vi "Test_PublishI32_SubBeforePub_OK.vi"(8 "error in (no error)":errorcluster, 11 "TestMediator In":refnum<class "TestMediationSemantics.lvclass">) -> (0 "error out":errorcluster, 3 "TestMediator Out":refnum<class "TestMediationSemantics.lvclass">)   [LabVIEW 2017, in "TestMediationSemantics.lvclass"]
uses:
  TestMediationSemantics.lvclass
  Source/Framework/Mediator/Mediator/Mediator.lvclass
  C:/Program Files (x86)/National Instruments/LabVIEW 2017/vi.lib/ActorFramework/Actor/Actor.lvclass
  Source/Framework/IMediator/PublishRequest/PublishRequest.lvclass/PublishRequest.ctl
  Source/Framework/SubscriptionPolicy/BasicSubscription/BasicSubscription.lvclass/BasicSubscription.ctl
  Source/Framework/IMediator/SubscriptionRequest/SubscriptionRequest.lvclass/SubscriptionRequest.ctl
  Source/Framework/IMediator/IMediator Messages/Subscribe Msg/Subscribe Msg.lvclass/Subscribe Msg.ctl
  <vilib>/ActorFramework/Message Enqueuer/Message Enqueuer.lvclass/Message Enqueuer.ctl
  Source/Framework/IMediator/IMediator Messages/Publish Msg/Publish Msg.lvclass/Publish Msg.ctl
  gpm_packages/@cs/transport/Source/Concrete/QueueTransport/QueueTransport.lvclass/QueueTransport.ctl
  <vilib>/ActorFramework/Message Enqueuer/Enqueue.vi
  Source/Framework/SubscriptionPolicy/BasicSubscription/BasicSubscription.lvclass
  C:/Git/mva-framework/Source/Framework/IMediator/ISubscriptionPolicy/ISubscriptionPolicy.lvclass
  gpm_packages/@cs/transport/Source/Concrete/QueueTransport/QueueTransport.lvclass
  C:/Git/mva-framework/gpm_packages/@cs/transport/Source/ITransport/ITransport.lvclass
  Source/Framework/IMediator/IMediator Messages/Subscribe Msg/Subscribe Msg.lvclass
  C:/Program Files (x86)/National Instruments/LabVIEW 2017/vi.lib/ActorFramework/Message/Message.lvclass
  Source/Framework/IMediator/IMediator Messages/Publish Msg/Publish Msg.lvclass
  <vilib>/ActorFramework/Stop Msg/Stop Msg.lvclass
  <vilib>/ActorFramework/Message Priority Queue/Priority Enqueue.vi
  <vilib>/Utility/error.llb/Error Cluster From Error Code.vi
  Source/Framework/IMediator/SubscriptionRequest/SubscriptionRequest.lvclass
  Source/Framework/IMediator/PublishRequest/PublishRequest.lvclass
  <vilib>/ActorFramework/Actor/Actor.lvclass
  Source/Framework/IMediator/ISubscriptionPolicy/ISubscriptionPolicy.lvclass
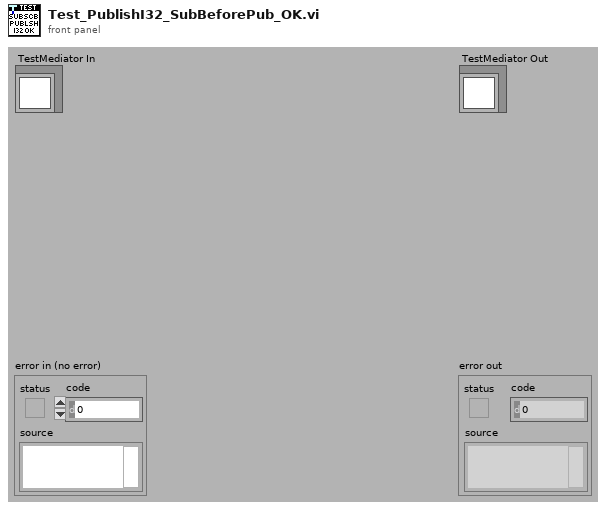
[diagram p1: front panel]
types:
  T1 = typedef "IMediator.lvlib/ISubscriptionPolicy.lvclass/ISubscriptionPolicy Reference.ctl" = refnum<data-value>
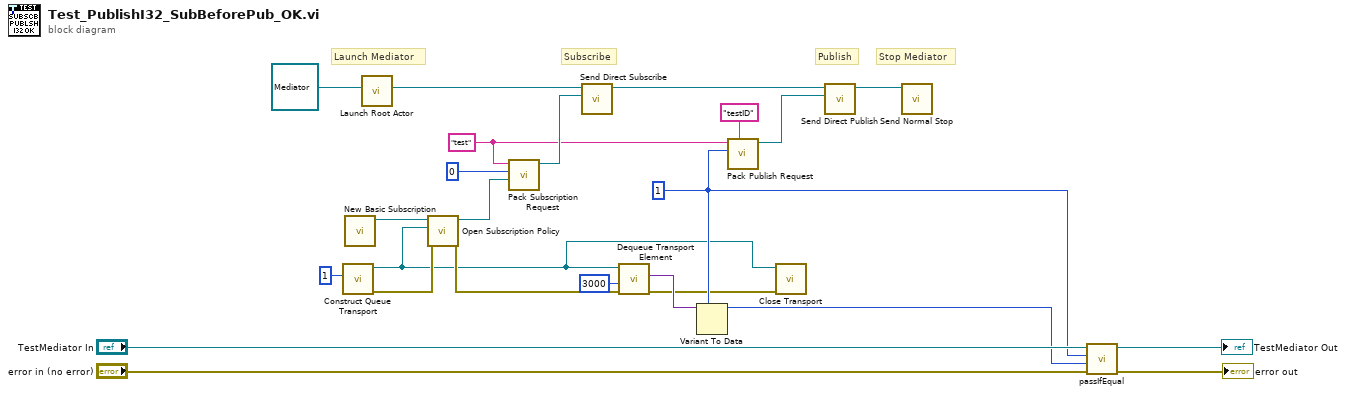
[diagram p0: block diagram]
diagram:
  w5 = "test" ("Datum Name")
  w4 = 1
  # "Launch Mediator"
  # "Stop Mediator"
  # "Subscribe"
  # "Publish"
  n1 = call "Construct Queue Transport.vi"("Max Queue Size (-1)"=1) -> ("error out"=w15:errorcluster, "QueueTransport"=w2:refnum<class "QueueTransport.lvclass">)  [unwired: 9 in]
  n2 = call "New Basic Subscription.vi"() -> ("BasicSubscription Out"=w11:refnum<class "BasicSubscription.lvclass">)  [unwired: 11 in]
  n3 = call <vilib>:"Launch Root Actor.vi"("Actor"=refnum<class "Mediator.lvclass"> refnum ("Mediator.lvlib:Mediator.lvclass")) -> ("Actor's Enqueuer"=w8:refnum<class "Message Enqueuer.lvclass">)  [unwired: 9 in, 1 out]
  n4 = call "Open Subscription Policy.vi"("error in (no error)"=w15, "Transport"=w2, "SubscriptionPolicy"=w11) -> ("error out"=w14:errorcluster, "Subscription Policy"=w7:T1)  [unwired: 7 in]
  n5 = call "Pack Subscription Request.vi"("Subscription Policy"=w7, "Type"=0, "Datum Name"=w5) -> ("SubscriptionRequest"=w19:refnum<class "SubscriptionRequest.lvclass">)  [unwired: 8 in]
  n6 = call "Send Direct Subscribe.vi"("Subscription Request"=w19, "Message Enqueuer"=w8) -> ("Message Enqueuer out"=w10:refnum<class "Message Enqueuer.lvclass">)  [unwired: 8 in, 1 out]
  n7 = call "Dequeue Transport Element.vi"("error in (no error)"=w14, "Timeout In ms (-1)"=3000, "QueueTransport"=w2) -> ("error out"=w1:errorcluster, "Data"=w13:variant)  [unwired: 5 in, 2 out]
  n8 = Variant To Data(type=w4, Variant=w13) -> (data=w12:i32)  [unwired: 1 in, 1 out]
  n9 = call "Pack Publish Request.vi"("Publisher ID"="testID", "Data to Publish"=w4, "Datum Name"=w5) -> ("PublishRequest"=w3:refnum<class "PublishRequest.lvclass">)  [unwired: 8 in]
  n10 = call-dynamic "Close Transport.vi"("error in (no error)"=w1, "QueueTransport"=w2) -> ()  [unwired: 9 in, 1 out]
  n11 = call "Send Direct Publish.vi"("PublishRequest"=w3, "Mediator Enqeuer"=w10) -> ("Mediator Enqueuer out"=w9:refnum<class "Message Enqueuer.lvclass">)  [unwired: 8 in, 1 out]
  n12 = call <vilib>:"Send Normal Stop.vi"("Message Enqueuer"=w9) -> ()  [unwired: 10 in, 1 out]
  n13 = call-dynamic "passIfEqual.vi"("error in (no error)"="error in (no error)", "y"=w12, "x"=w4, "TestCase in"="TestMediator In") -> ("error out"=→"error out":errorcluster, "TestCase out"=→"TestMediator Out":refnum<class "TestMediationSemantics.lvclass">)  [unwired: 6 in]
